vi "main.vi"() -> ()   [LabVIEW 2026, in "Server Controller.lvlib" / "Server Controller.lvclass"]
uses:
  Server Controller.lvclass
  UI/Server UI.lvclass
  Server Config.lvclass
  Server Controller.lvclass/Server Controller.ctl
  MAL-Framework/user.lib/Common Components/Controller/Controller.lvclass
  <vilib>/ActorFramework/Actor/Actor.lvclass
panel:
  out "Path to config file":path
  in  "Cancel Button":bool
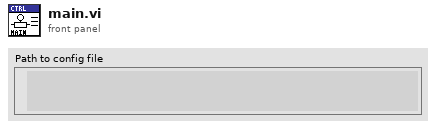
[diagram p1: front panel]
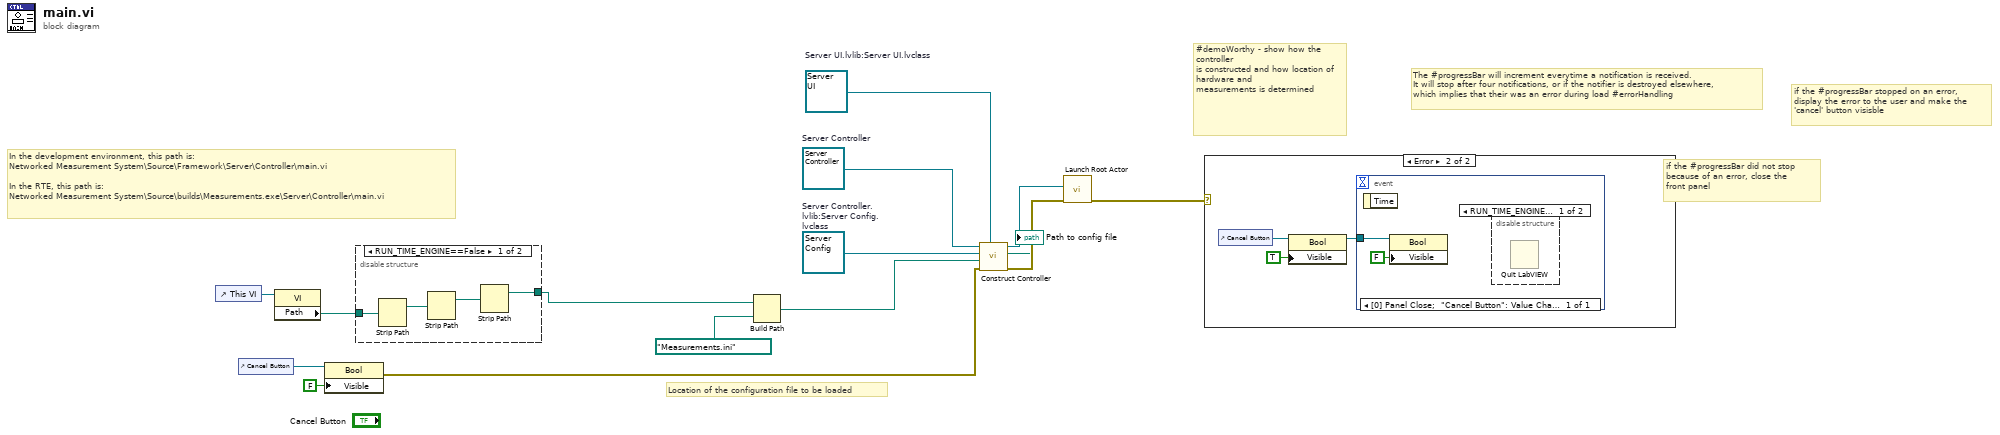
[diagram p0: block diagram]
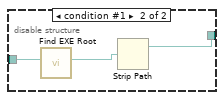
[diagram p2: hidden frame]
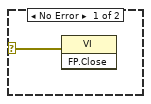
[diagram p3: hidden frame]
diagram:
  w7 = refnum<class "Server Config.lvclass"> refnum  # Server Controller.lvlib:Server Config.lvclass
  w6 = refnum<class "Server UI.lvclass"> refnum  # Server UI.lvlib:Server UI.lvclass
  w5 = refnum<class "Server Controller.lvclass"> refnum  # Server Controller
  # "Location of the configuration file to be loaded"
  # "In the development environment, this path is: \nNetworked Measurement System\\Source\\Framework\\Server\\Controller\\main.vi\n\nIn the RTE, this path is:\nNetworked Measurement System\\Source\\builds\\Measurements.exe\\Server\\Controller\\main.vi"
  # "#demoWorthy - show how the controller \nis constructed and how location of hardware and \nmeasurements is determined"
  # "if the #progressBar stopped on an error,\ndisplay the error to the user and make the\n'cancel' button visisble"
  # "if the #progressBar did not stop\nbecause of an error, close the \nfront panel"
  # "The #progressBar will increment everytime a notification is received.\nIt will stop after four notifications, or if the notifier is destroyed elsewhere,\nwhich implies that their was an error during load #errorHandling"
  n1 = control-ref of="This VI"() -> (w13:refnum<vi>)
  n2 = control-ref of="Cancel Button"() -> (w15:refnum<vi>)
  n3 = property class="VI"(reference=w13) -> ("Path"=w12:path)  [unwired: 1 in, 2 out]
  n4 = property class="Bool"(reference=w15, "Visible"=FALSE) -> (error out=w3:errorcluster)  [unwired: 1 in, 1 out]
  n5 = disable-structure shown="RUN_TIME_ENGINE==False" {
    disable-tunnel: w12 -> [w18 w22]
    disable-tunnel: [w16 w20] -> w9
    frame condition #0 (active) {
      n6 = Strip Path(path=w18) -> (stripped path=w19:path)  [unwired: 1 out]
      n7 = Strip Path(path=w19) -> (stripped path=w17:path)  [unwired: 1 out]
      n8 = Strip Path(path=w17) -> (stripped path=w16:path)  [unwired: 1 out]
    }
    frame condition #1 {
      n9 = call "Find EXE Root.vi"("Path"=w22) -> ("Location of EXE"=w21:path)  [unwired: 10 in]
      n10 = Strip Path(path=w21) -> (stripped path=w20:path)  [unwired: 1 out]
    }
  }
  n11 = Build Path(base path=w9, name or relative path=path "Measurements.ini" ("VI Path")) -> (appended path=w8:path)
  n12 = call "Construct Controller.vi"("UI.lvclass"=w6, "error in (no error)"=w3, "Root Path"=w8, "Configuration.lvlib:Configuration.lvclass"=w7, "Controller Actor.lvlib:Controller.lvclass"=w5) -> ("error out"=w2:errorcluster, "Path to config file"=→"Path to config file":path, "Controller Actor.lvlib:Controller.lvclass 2"=w4:refnum<class "Server Controller.lvclass">)  [unwired: 4 in]
  n13 = call <vilib>:"Launch Root Actor.vi"("error in (no error)"=w2, "Actor"=w4) -> ("error out"=w11:errorcluster)  [unwired: 8 in, 1 out]
  n14 = case shown="Error" w11 {
    selector: w11 -> [w23 _]
    frame No Error {
      n15 = invoke class="VI" method="FP.Close"(error in=w23) -> ()  [unwired: 2 in, 3 out]
    }
    frame Error {
      n16 = control-ref of="Cancel Button"() -> (w25:refnum<vi>)
      n17 = property class="Bool"(reference=w25, "Visible"=TRUE) -> (reference out=w24:refnum<vi>)  [unwired: 1 in, 1 out]
      n18 = event shown="[0] Panel Close;  \"Cancel Button\": Value Change" {
        selector: _ -> [_]
        dyn-events: _ -> [_]
        timeout: _ -> [_]
        tunnel: w24 -> [w28]
        event Panel Close; "Cancel Button": Value Change {
          n19 = event-data() -> ()  [unwired: 1 in, 1 out]
          n20 = property class="Bool"(reference=w28, "Visible"=FALSE) -> ()  [unwired: 1 in, 2 out]
          n21 = disable-structure shown="RUN_TIME_ENGINE==True" {
            frame condition #0 {
              n22 = Quit LabVIEW() -> ()  [unwired: 1 in]
            }
            frame condition #1 (active) {
            }
          }
        }
      }
    }
  }
